vi "Initialize Transfers.vi"(8 "error in (no error)":errorcluster, 11 "Group Configuration":refnum<class "Group Configuration.lvclass">) -> (0 "error out":errorcluster, 2 "max buffer size":u64, 3 "transfer parameters":T1[](array[typedef]))   [LabVIEW 2017, in "UDP Transceiver.lvlib" / "UDP Transceiver.lvclass"]
uses:
  UDP Transceiver.lvclass
  Transfer Parameters.ctl
  DSF Core.lvlibp/Classes/Configuration/Core/Group/Group Configuration.lvclass
  Throw Unknown Setting Error.vi
  DSF Core.lvlibp/Classes/Configuration/Core/Transfer/Transfer Configuration.lvclass
  DSF Core.lvlibp/Classes/Configuration Session/Configuration Session.lvclass
  DSF Core.lvlibp/Classes/Configuration/Core/Core Configuration.lvclass
  C:/Git/DSF/Components/DSF Core.lvlibp/Classes/Configuration/Core/Core Configuration.lvclass
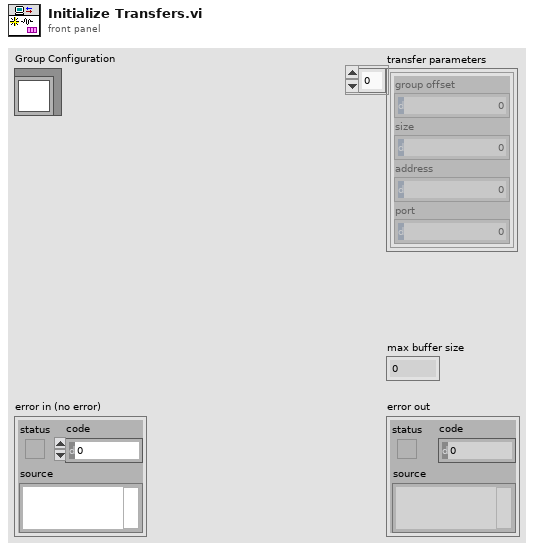
[diagram p1: front panel]
types:
  T1 = typedef "UDP Transceiver.lvlib/UDP Transceiver.lvclass/Transfer Parameters.ctl" = cluster{"group offset":u64, "size":u64, "address":u32, "port":u16}
  T2 = typedef "DSF Core.lvlibp/Group Configuration.lvclass/Core Group Configuration.ctl" = cluster{"name":string, "direction":T3, "cycle timing":T4, "timeout behavior":T5, "enable conversion":bool}
  T3 = typedef "DSF Core.lvlibp/DSF Direction.ctl" = enum8{"Tx", "Rx"}
  T4 = typedef "DSF Core.lvlibp/DSF Timing Info.ctl" = cluster{"priority":u64, "decimation":u64, "offset":u64}
  T5 = typedef "DSF Core.lvlibp/DSF Timeout Behavior.ctl" = enum8{"Increment Late Count", "Throw Error"}
  T6 = typedef "DSF Core.lvlibp/DSF Settings Info.ctl" = cluster{"component":string, "values":cluster{"key":string, "value":string}[]}
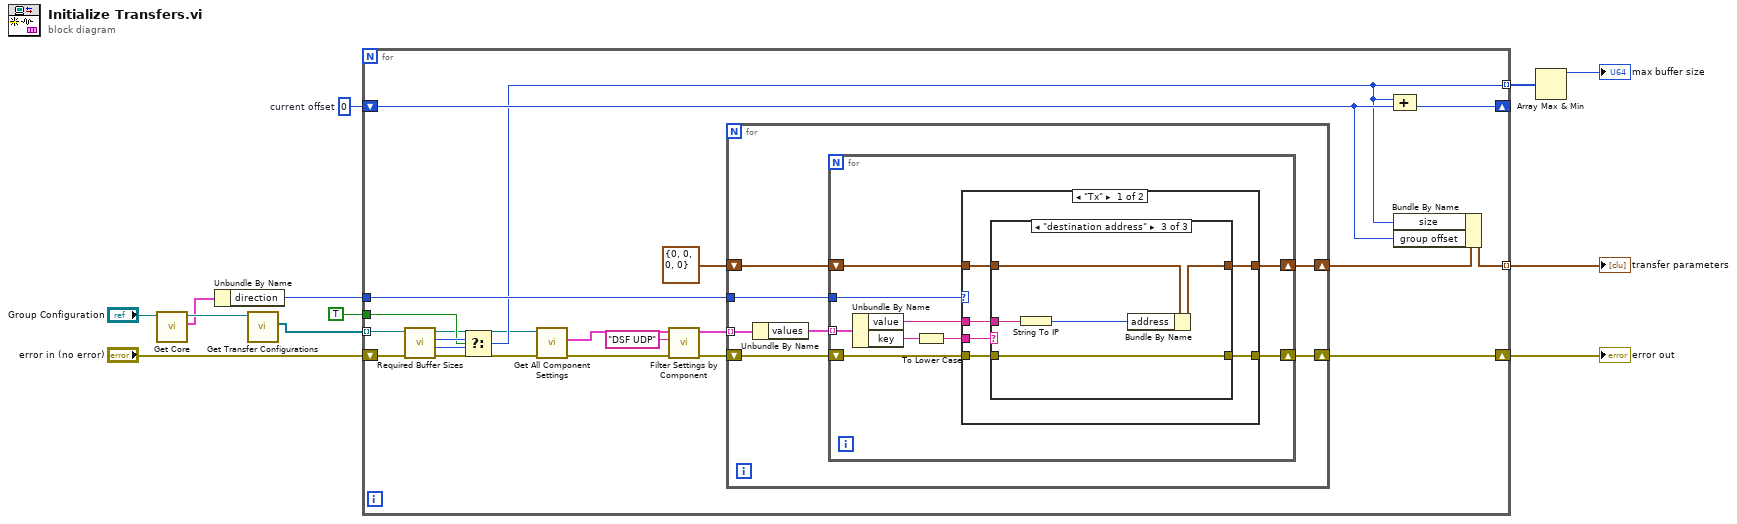
[diagram p0: block diagram]
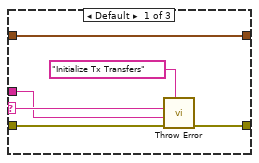
[diagram p2: hidden frame]
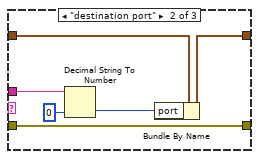
[diagram p3: hidden frame]
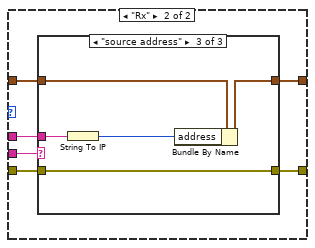
[diagram p4: hidden frame]
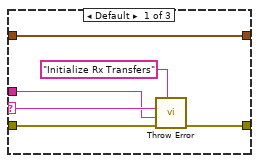
[diagram p5: hidden frame]
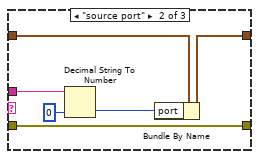
[diagram p6: hidden frame]
diagram:
  w6 = u64 0  # current offset
  n1 = call "Get Core.vi"("Group Configuration in"="Group Configuration") -> ("core"=w3:T2, "Group Configuration out"=w4:refnum<class "Group Configuration.lvclass">)  [unwired: 8 in, 1 out]
  n2 = Unbundle By Name(w3) -> ("direction"=w7:T3)
  n3 = call "Get Transfer Configurations.vi"("Group Configuration in"=w4) -> ("Transfer Configurations"=w2:refnum<class "Transfer Configuration.lvclass">[])  [unwired: 8 in, 2 out]
  n4 = for {
    shift-right: [w32] -> w10
    shift-left: "error in (no error)" -> [w16]
    tunnel: w2 -> [w31] mode=indexing
    tunnel: [w18] -> w11 mode=indexing
    tunnel: [w20] -> w9 mode=indexing
    tunnel: TRUE -> [w23]
    tunnel: w7 -> [w25]
    shift-right: [w22] -> _
    shift-left: w6 -> [w21]
    n5 = call-dynamic "Required Buffer Sizes.vi"("error in (no error)"=w16, "Transfer Configuration in"=w31) -> ("error out"=w15:errorcluster, "string size"=w24:u64, "engine size"=w27:u64, "Transfer Configuration out"=w17:refnum<class "Transfer Configuration.lvclass">)  [unwired: 6 in]
    n6 = Select(t=w27, s=w23, f=w24) -> (s? t:f=w20:u64)
    n7 = call "Get All Component Settings.vi"("error in (no error)"=w15, "Runtime Configuration in"=w17) -> ("error out"=w13:errorcluster, "component settings"=w14:T6[])  [unwired: 7 in, 1 out]
    n8 = call "Filter Settings by Component.vi"("error in (no error)"=w13, "component"="DSF UDP", "settings"=w14) -> ("error out"=w30:errorcluster, "filtered settings"=w28:T6[])  [unwired: 7 in]
    n9 = for {
      tunnel: w28 -> [w35] mode=indexing
      shift-right: [w37] -> w19
      shift-left: T1 {"group offset"=0, "size"=0, "address"=0, "port"=0} ("Transfer Tx") -> [w38]
      shift-right: [w39] -> w32
      shift-left: w30 -> [w36]
      tunnel: w25 -> [w33]
      n10 = Unbundle By Name(w35) -> ("values"=w34:cluster{"key":string, "value":string}[])
      n11 = for {
        tunnel: w34 -> [w48] mode=indexing
        shift-right: [w43] -> w39
        shift-left: w36 -> [w47]
        shift-right: [w45] -> w37
        shift-left: w38 -> [w46]
        tunnel: w33 -> [w40]
        n12 = Unbundle By Name(w48) -> ("value"=w44:string, "key"=w42:string)
        n13 = To Lower Case(string=w42) -> (all lower case string=w41:string)
        n14 = case shown="\"Tx\"" w40 {
          tunnel: w47 -> [w54 w77]
          tunnel: w46 -> [w53 w74]
          tunnel: [w52 w73] -> w45
          tunnel: w44 -> [w51 w75]
          tunnel: [w50 w72] -> w43
          tunnel: w41 -> [w49 w76]
          frame "Tx" {
            n15 = case shown="\"destination address\"" w49 {
              selector: w49 -> [w56 _ _]
              tunnel: w51 -> [w55 w66 w70]
              tunnel: w54 -> [w58 w63 w71]
              tunnel: [w57 w63 w71] -> w50
              tunnel: w53 -> [w60 w62 w67]
              tunnel: [w60 w61 w68] -> w52
              frame Default {
                n16 = call-poly "Throw Error.vi"("source vi name"="Initialize Tx Transfers", "error in (no error)"=w58, "value"=w55, "key"=w56) -> ("error out"=w57:errorcluster)  [unwired: 7 in]
              }
              frame "destination port" {
                n17 = Decimal String To Number(string=w66, default (0L)=u16 0 ("default (0 I32)")) -> (number=w64:u16)  [unwired: 1 in, 1 out]
                n18 = Bundle By Name(cluster=w62, "port"=w64) -> (w61:T1)
              }
              frame "destination address" {
                n19 = String To IP(1:w70) -> (0:w69:u32)
                n20 = Bundle By Name(cluster=w67, "address"=w69) -> (w68:T1)
              }
            }
          }
          frame "Rx" {
            n21 = case shown="\"source address\"" w76 {
              selector: w76 -> [w79 _ _]
              tunnel: w75 -> [w78 w89 w91]
              tunnel: w77 -> [w82 w86 w94]
              tunnel: [w81 w86 w94] -> w72
              tunnel: w74 -> [w80 w85 w93]
              tunnel: [w80 w84 w92] -> w73
              frame Default {
                n22 = call-poly "Throw Error.vi"("source vi name"="Initialize Rx Transfers", "error in (no error)"=w82, "value"=w78, "key"=w79) -> ("error out"=w81:errorcluster)  [unwired: 7 in]
              }
              frame "source port" {
                n23 = Decimal String To Number(string=w89, default (0L)=u16 0 ("default (0 I32)")) -> (number=w87:u16)  [unwired: 1 in, 1 out]
                n24 = Bundle By Name(cluster=w85, "port"=w87) -> (w84:T1)
              }
              frame "source address" {
                n25 = String To IP(1:w91) -> (0:w90:u32)
                n26 = Bundle By Name(cluster=w93, "address"=w90) -> (w92:T1)
              }
            }
          }
        }
      }
    }
    n27 = Compound Arithmetic op=ADD(w20, w21) -> (w22:u64)
    n28 = Bundle By Name(cluster=w19, "size"=w20, "group offset"=w21) -> (w18:T1)
  }
  "error out" <- w10
  "transfer parameters" <- w11
  n29 = Array Max & Min(array=w9) -> (max value=→"max buffer size":u64)  [unwired: 3 out]
